vi "element_editor_load_vali.vi"(6 "LUA Validation File":path, 10 "Parameters Tree":refnum<vi>) -> (2 "Vali File Loaded":bool)   [LabVIEW 2019]
uses:
  lib/libSpecValiReader/libSpecValiReader.lvlib
panel:
  # "*******************************************************************\nBiogas Plant Control\n\nAuthor: Paul Zügel\nGCSC-Frankfurt am Main 2020\n\n*******************************************************************"
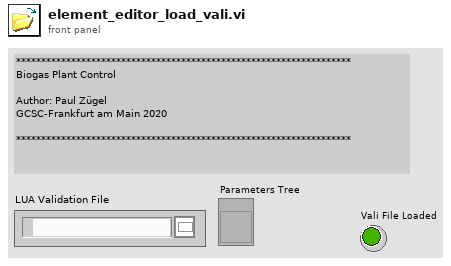
[diagram p1: front panel]
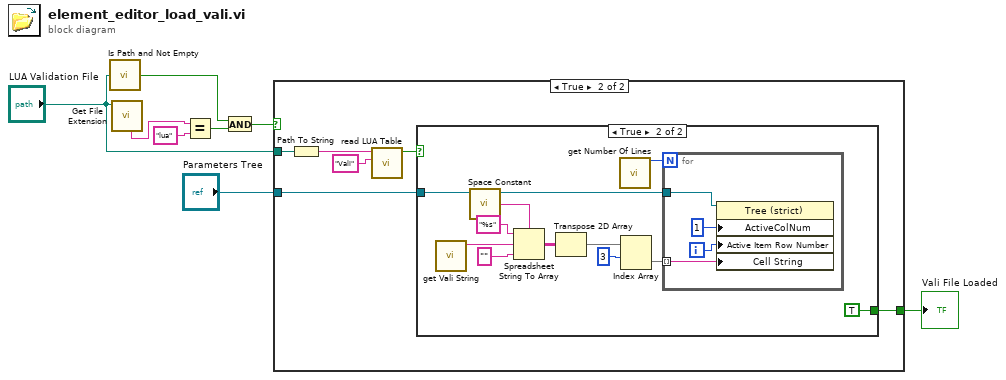
[diagram p0: block diagram]
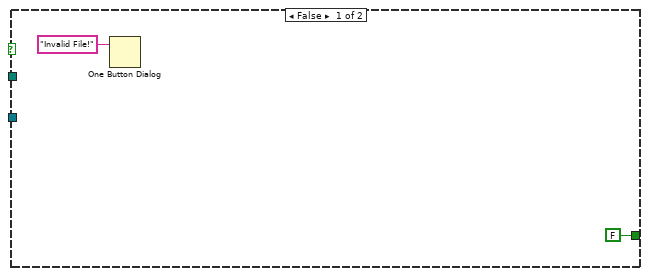
[diagram p2: hidden frame]
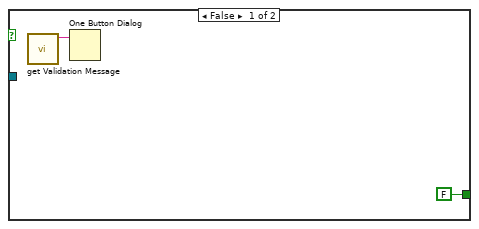
[diagram p3: hidden frame]
diagram:
  n1 = call <vilib>:"Is Path and Not Empty.vi"("path"="LUA Validation File") -> ("Is Path and Not Empty?"=w4:bool)  [unwired: 4 in]
  n2 = call <vilib>:"Get File Extension.vi"("file"="LUA Validation File") -> ("unmodified file extension"=w7:string)  [unwired: 6 in, 4 out]
  n3 = Equal?(x=w7, y="lua") -> (x = y?=w3:bool)
  n4 = And(x=w4, y=w3) -> (x .and. y?=w2:bool)
  n5 = case shown="True" w2 {
    tunnel: "Parameters Tree" -> [_ w15]
    tunnel: "LUA Validation File" -> [_ w16]
    tunnel: [FALSE ("Vali File Loaded") w11] -> w1
    frame False {
      n6 = One Button Dialog(message="Invalid File!") -> ()  [unwired: 1 in, 1 out]
    }
    frame True {
      n7 = Path To String(path=w16) -> (string=w13:string)
      n8 = call "read LUA Table.vi"("vali_or_spec"="Vali" ("spec_filename"), "filename"=w13) -> ("function return"=w12:bool)  [unwired: 8 in, 1 out]
      n9 = case shown="True" w12 {
        tunnel: w15 -> [_ w28]
        tunnel: [FALSE ("Vali File Loaded") TRUE ("Vali File Loaded")] -> w11
        frame False {
          n10 = call "get Validation Message.vi"() -> ("function return"=w18:string)  [unwired: 10 in, 1 out]
          n11 = One Button Dialog(message=w18) -> ()  [unwired: 1 in, 1 out]
        }
        frame True {
          n12 = call "get Vali String.vi"() -> ("function return"=w23:string)  [unwired: 10 in, 1 out]
          n13 = call <vilib>:"Space Constant.vi"() -> ("String"=w24:string)
          n14 = Spreadsheet String To Array(delimiter (Tab)=w24, format string="%s", spreadsheet string=w23, array type (2D Dbl)="") -> (array=w22:string[][])
          n15 = Transpose 2D Array(2D array=w22) -> (transposed array=w21:string[][])
          n16 = call "get Number Of Lines.vi"() -> ("function return"=w29:i32)  [unwired: 10 in, 1 out]
          n17 = Index Array(array=w21, index (row)=3) -> (element=w27:string[])  [unwired: 1 in]
          n18 = for {
            N: w29 -> [_]
            tunnel: w28 -> [w31]
            tunnel: w27 -> [w30] mode=indexing
            i -> [w32]
            n19 = property on="Property Node" class="Tree (strict)"(reference=w31, "ActiveColNum"=1 ("Active Cell:Active Column Number"), "Active Item Row Number"=w32, "Cell String"=w30) -> ()  [unwired: 1 in, 2 out]
          }
        }
      }
    }
  }
  "Vali File Loaded" <- w1
